vi "MoAgSy_GPG_string2tmp.vi"(2 "String":string, 5 "error in (no error)":errorcluster) -> (16 "Path":path, 19 "error out":errorcluster)   [LabVIEW 2009, in "MoAgSy.lvlib" / "MoAgSy_GPG.lvclass"]
uses:
  MoAgSy_GPG.lvclass
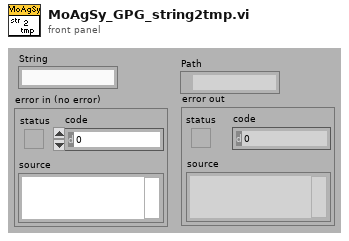
[diagram p1: front panel]
types:
  T1 = enum16{"open", "replace", "create", "open or create", "replace or create", "replace or create with confirmation"}
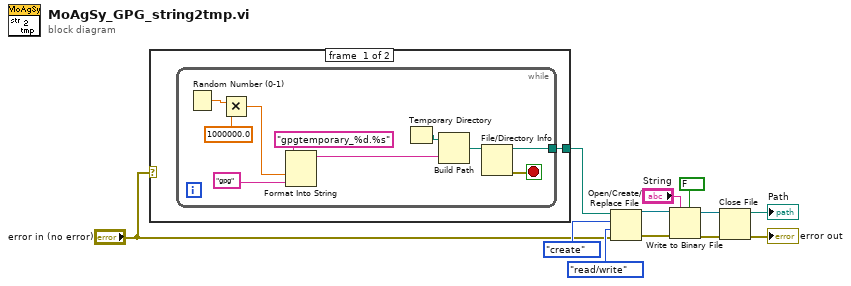
[diagram p0: block diagram]
diagram:
  n1 = case shown="No Error" "error in (no error)" {
    tunnel: [w13 _] -> w12
    frame #0 {
      n2 = while {
        tunnel: [w16] -> w13
        stop <- w17 stop-if-true
        n3 = Random Number (0-1)() -> (number: 0 to 1=w23:dbl)
        n4 = Multiply(x=w23, y=1000000.0) -> (x*y=w20:dbl)
        n5 = Format Into String(format string="gpgtemporary_%d.%s", w20, "gpg" ("input 2")) -> (resulting string=w19:string)  [unwired: 2 in, 1 out]
        n6 = Temporary Directory() -> (w14:path)
        n7 = Build Path(base path=w14, name or relative path=w19) -> (appended path=w18:path)
        n8 = File/Directory Info(path=w18) -> (path out=w16:path, error out=w17:errorcluster)  [unwired: 1 in, 5 out]
      }
    }
    frame #1 {
    }
  }
  n9 = Open/Create/Replace File(file path (use dialog)=w12, error in="error in (no error)", operation (0:open)=T1."create", access (0:read/write)=enum16{"read/write", "read-only", "write-only"}."read/write") -> (refnum out=w8:refnum<file>, error out=w6:errorcluster)  [unwired: 3 out]
  n10 = Write to Binary File(file (use dialog)=w8, data="String", error in=w6, 5:FALSE ("prepend array or string size? (T)")) -> (refnum out=w5:refnum<file>, error out=w4:errorcluster)  [unwired: 3 out]
  n11 = Close File(refnum=w5, error in=w4) -> (path=→"Path":path, error out=→"error out":errorcluster)
